vi "CTL_Set_Resistor Value.vi"(10 "Level IN inches":dbl, 11 "Spec Range":T1) -> (3 "Numeric":dbl)   [LabVIEW 2024]
uses:
  Control Definitions/Ded LUT_Status.ctl
  Control Definitions/Ded Spec RNG.ctl
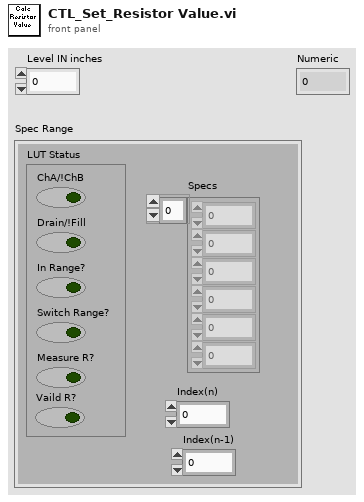
[diagram p1: front panel]
types:
  T1 = typedef "Ded Spec RNG.ctl" = cluster{"Specs":dbl[], "Index(n)":i32, "LUT Status":T2, "Index(n-1)":i32}
  T2 = typedef "Ded LUT_Status.ctl" = cluster{"ChA/!ChB":bool, "Drain/!Fill":bool, "In Range?":bool, "Switch Range?":bool, "Measure R?":bool, "Vaild R?":bool}
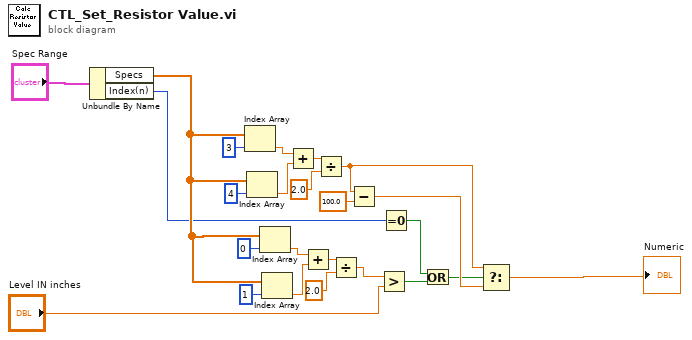
[diagram p0: block diagram]
diagram:
  n1 = Unbundle By Name("Spec Range") -> ("Specs"=w2:dbl[], "Index(n)"=w1:i32)
  n2 = Index Array(array=w2, index=3) -> (element=w10:dbl)
  n3 = Index Array(array=w2, index=4) -> (element=w11:dbl)
  n4 = Index Array(array=w2, index=0) -> (element=w16:dbl)
  n5 = Index Array(array=w2, index=1) -> (element=w17:dbl)
  n6 = Add(x=w10, y=w11) -> (x+y=w12:dbl)
  n7 = Add(x=w16, y=w17) -> (x+y=w18:dbl)
  n8 = Divide(x=w12, y=2.0) -> (x/y=w22:dbl)
  n9 = Divide(x=w18, y=2.0) -> (x/y=w20:dbl)
  n10 = Subtract(x=w22, y=100.0) -> (x-y=w24:dbl)
  n11 = Greater?(x=w20, y="Level IN inches") -> (0:w7:bool)
  n12 = Equal To 0?(x=w1) -> (x = 0?=w5:bool)
  n13 = Or(x=w5, y=w7) -> (x .or. y?=w6:bool)
  n14 = Select(t=w22, s=w6, f=w24) -> (s? t:f=→"Numeric":dbl)
